vi "Publish Current State.vi"(8 "error in (no error)":errorcluster, 10 "State":string, 11 "Process in":refnum<class "Process.lvclass">) -> (0 "error out":errorcluster, 3 "Process out":refnum<class "Process.lvclass">)   [LabVIEW 2019, in "TimingDRV Engine.lvlib" / "Process.lvclass"]
uses:
  Process.lvclass
  Process.lvclass/Process.ctl
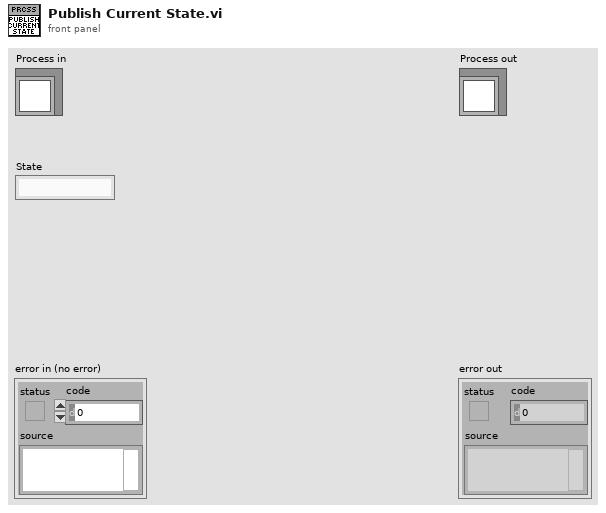
[diagram p1: front panel]
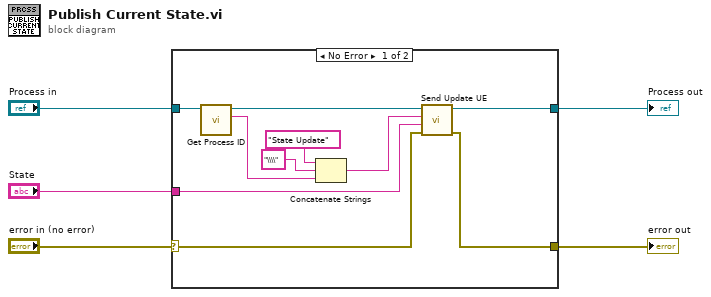
[diagram p0: block diagram]
diagram:
  n1 = case shown="No Error" "error in (no error)" {
    selector: "error in (no error)" -> [w11 w17]
    tunnel: [w10 w17] -> w4
    tunnel: [w12 w16] -> w2
    tunnel: "Process in" -> [w13 w16]
    tunnel: "State" -> [w9 _]
    frame No Error {
      n2 = call "Get Process ID.vi"("CD_Process in"=w13) -> ("Process ID"=w6:string, "CD_Process out"=w14:refnum<class "Process.lvclass">)  [unwired: 9 in]
      n3 = Concatenate Strings("State Update" ("State"), "\\\\" ("string"), w6) -> (w15:string)
      n4 = call "Send Update UE.vi"("error in (no error)"=w11, "Payload"=w9, "Update Message"=w15, "Process in"=w14) -> ("error out"=w10:errorcluster, "Process out"=w12:refnum<class "Process.lvclass">)  [unwired: 6 in]
    }
    frame Error {
    }
  }
  "error out" <- w4
  "Process out" <- w2
